vi "Code Conversion Paths.vi"(11 "error in (no error)":errorcluster) -> (2 "Folders to Ignore":path, 3 "Deafult value setter VI":path, 4 "IS Project Directory":path, 6 "IO Controls":path, 8 "Get Resource VI":path, 10 "Error Log Path":path, 13 "Deserializer":path, 14 "Serializer":path, 15 "error out":errorcluster)   [LabVIEW 2021, in "Path Functions.lvlib"]
uses:
  Path Functions.lvlib
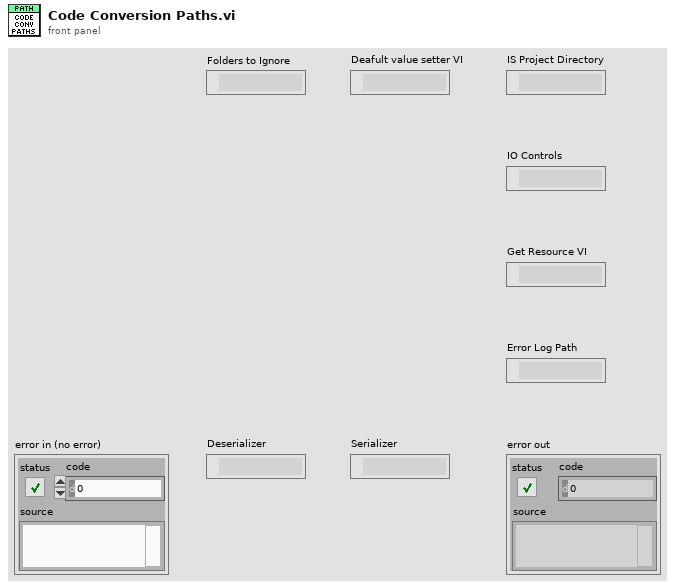
[diagram p1: front panel]
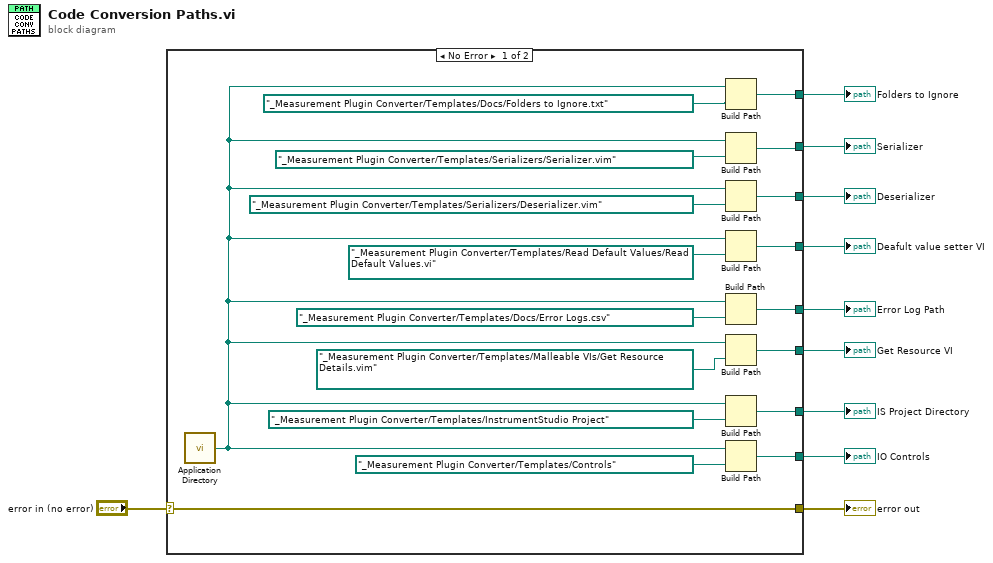
[diagram p0: block diagram]
diagram:
  n1 = case shown="No Error" "error in (no error)" {
    selector: "error in (no error)" -> [w23 w29]
    tunnel: [w28 _] -> w10
    tunnel: [w27 _] -> w9
    tunnel: [w26 _] -> w8
    tunnel: [w24 _] -> w7
    tunnel: [w17 _] -> w6
    tunnel: [w23 w29] -> w5
    tunnel: [w20 _] -> w4
    tunnel: [w18 _] -> w3
    tunnel: [w14 _] -> w2
    frame No Error {
      n2 = call <vilib>:"Application Directory.vi"() -> ("Application Directory"=w16:path)
      n3 = Build Path(base path=w16, name or relative path=path "_Measurement Plugin Converter/Templates/Docs/Folders to Ignore.txt") -> (appended path=w14:path)
      n4 = Build Path(base path=w16, name or relative path=path "_Measurement Plugin Converter/Templates/Serializers/Serializer.vim") -> (appended path=w17:path)
      n5 = Build Path(base path=w16, name or relative path=path "_Measurement Plugin Converter/Templates/Serializers/Deserializer.vim") -> (appended path=w20:path)
      n6 = Build Path(base path=w16, name or relative path=path "_Measurement Plugin Converter/Templates/Read Default Values/Read Default Values.vi") -> (appended path=w18:path)
      n7 = Build Path(base path=w16, name or relative path=path "_Measurement Plugin Converter/Templates/Docs/Error Logs.csv") -> (appended path=w24:path)
      n8 = Build Path(base path=w16, name or relative path=path "_Measurement Plugin Converter/Templates/Malleable VIs/Get Resource Details.vim") -> (appended path=w26:path)
      n9 = Build Path(base path=w16, name or relative path=path "_Measurement Plugin Converter/Templates/InstrumentStudio Project") -> (appended path=w28:path)
      n10 = Build Path(base path=w16, name or relative path=path "_Measurement Plugin Converter/Templates/Controls") -> (appended path=w27:path)
    }
    frame Error {
    }
  }
  "error out" <- w5
  "IS Project Directory" <- w10
  "IO Controls" <- w9
  "Get Resource VI" <- w8
  "Error Log Path" <- w7
  "Deserializer" <- w4
  "Serializer" <- w6
  "Deafult value setter VI" <- w3
  "Folders to Ignore" <- w2
